vi "Add Protection.vi"(8 "error in (no error)":errorcluster, 9 "Pad":bool, 10 "String in":string, 11 "Checksum U8 in":refnum<class "Checksum U8.lvclass">) -> (0 "error out":errorcluster, 2 "String out":string, 3 "Checksum U8 out":refnum<class "Checksum U8.lvclass">)   [LabVIEW 2023, in "Protections.lvlib" / "Checksum U8.lvclass"]
uses:
  Checksum U8.lvclass
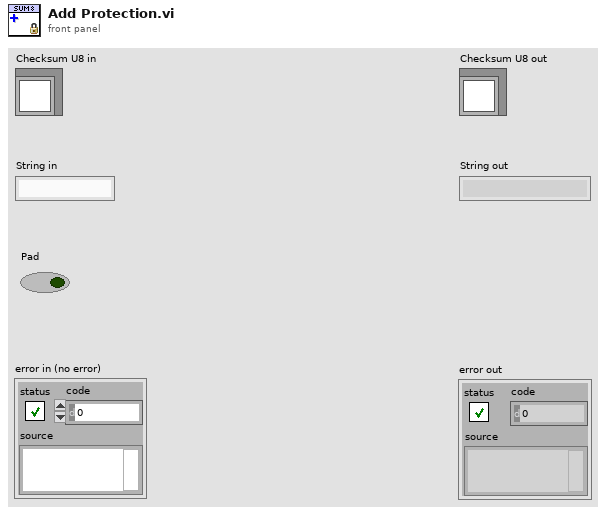
[diagram p1: front panel]
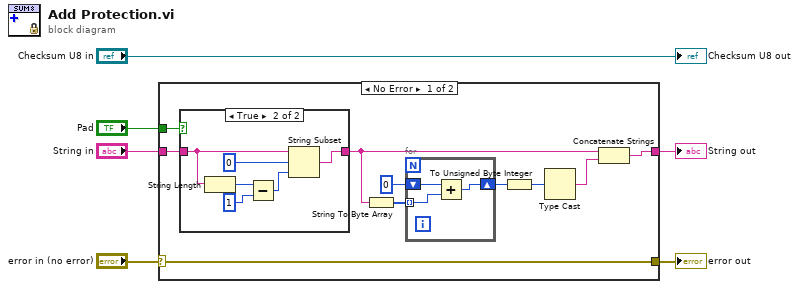
[diagram p0: block diagram]
diagram:
  n1 = case shown="No Error" "error in (no error)" {
    selector: "error in (no error)" -> [w10 w28]
    tunnel: "Pad" -> [w8 _]
    tunnel: "String in" -> [w9 w27]
    tunnel: [w11 w27] -> w3
    tunnel: [w10 w28] -> w1
    frame No Error {
      n2 = case shown="True" w8 {
        tunnel: w9 -> [w17 w23]
        tunnel: [w17 w18] -> w7
        frame False {
        }
        frame True {
          n3 = String Length(string=w23) -> (length=w21:i32)
          n4 = Subtract(x=w21, y=1) -> (x-y=w19:i32)
          n5 = String Subset(string=w23, offset (0)=0, length (rest)=w19) -> (substring=w18:string)
        }
      }
      n6 = String To Byte Array(string=w7) -> (unsigned byte array=w16:u8[])
      n7 = for {
        tunnel: w16 -> [w26] mode=indexing
        shift-right: [w24] -> w14
        shift-left: u64 0 -> [w25]
        n8 = Add(x=w25, y=w26) -> (x+y=w24:u64)
      }
      n9 = To Unsigned Byte Integer(number=w14) -> (unsigned 8bit integer=w12:u8)
      n10 = Type Cast(x=w12) -> (*(type *) &x=w13:string)  [unwired: 1 in]
      n11 = Concatenate Strings(w7, w13) -> (w11:string)
    }
    frame Error {
    }
  }
  "error out" <- w1
  "String out" <- w3
  "Checksum U8 out" <- "Checksum U8 in"
